vi "POSITION ARMS.vi"(6 "arm angle table":T1) -> ()   [LabVIEW 2020]
uses:
  Robot Global Data.vi
  <vilib>/Rock Robotics/Network Tables/NT Read Number.vi
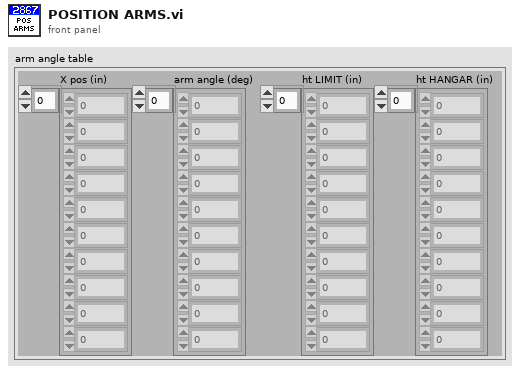
[diagram p1: front panel]
types:
  T1 = cluster{"X pos (in)":dbl[], "arm angle (deg)":dbl[], "ht LIMIT (in)":dbl[], "ht HANGAR (in)":dbl[]}
  T2 = cluster{"MIN":dbl, "MAX":dbl, "convert climber inches to tics":dbl}
  T3 = cluster{"MIN":dbl, "MAX":dbl, "convert arm inches to revs":dbl}
  T4 = typedef "WPI_MotorControlDeviceRef.ctl" = cluster{"DeviceStatus":errorcluster, "Type":T5, "PWM":cluster{"PWM Channel":T6, "DeadBand":T7}, "CAN":cluster{"Device Number":u8, "SetOutput VI Ref":variant, "GetOutput VI Ref":variant, "Enable VI Ref":variant, "Disable VI Ref":variant, "Data":variant}, "Invert":bool, "DIO PWM":cluster{"PWM \"Enable\" Channel":T6, "DIOChannel":T8, "PWM Rate":dbl}}
  T5 = typedef "WPI_MotorControlType.ctl" = enum16{"PWM", "CAN", "DIO PWM"}
  T6 = typedef "FPGA_DIOPWMChannel.ctl" = enum8{"PWM 0", "PWM 1", "PWM 2", "PWM 3", "PWM 4", "PWM 5", "PWM 6", "PWM 7", "PWM 8", "PWM 9", "PWM MXP 0", "PWM MXP 1", "PWM MXP 2", "PWM MXP 3", "PWM MXP 4", "PWM MXP 5", "PWM MXP 6", "PWM MXP 7", "PWM MXP 8", "PWM MXP 9", "Invalid"}
  T7 = typedef "WPI_PWMDeadband.ctl" = cluster{"Name":string, "maxPositivePwm":i32, "minPositivePwm":i32, "centerPwm":i32, "maxNegativePwm":i32, "minNegativePwm":i32, "angularRange":u16}
  T8 = typedef "FPGA_DIOChannel.ctl" = enum8{"DIO 0", "DIO 1", "DIO 2", "DIO 3", "DIO 4", "DIO 5", "DIO 6", "DIO 7", "DIO 8", "DIO 9", "DIO MXP 0", "DIO MXP 1", "DIO MXP 2", "DIO MXP 3", "DIO MXP 4", "DIO MXP 5", "DIO MXP 6", "DIO MXP 7", "DIO MXP 8", "DIO MXP 9", "DIO MXP 10", "DIO MXP 11", "DIO MXP 12", "DIO MXP 13", "DIO MXP 14", "DIO MXP 15", "SPI Port CS1", "SPI Port CS2", "SPI Port CS3", "SPI Port MISO", "SPI Port MOSI", "Invalid"}
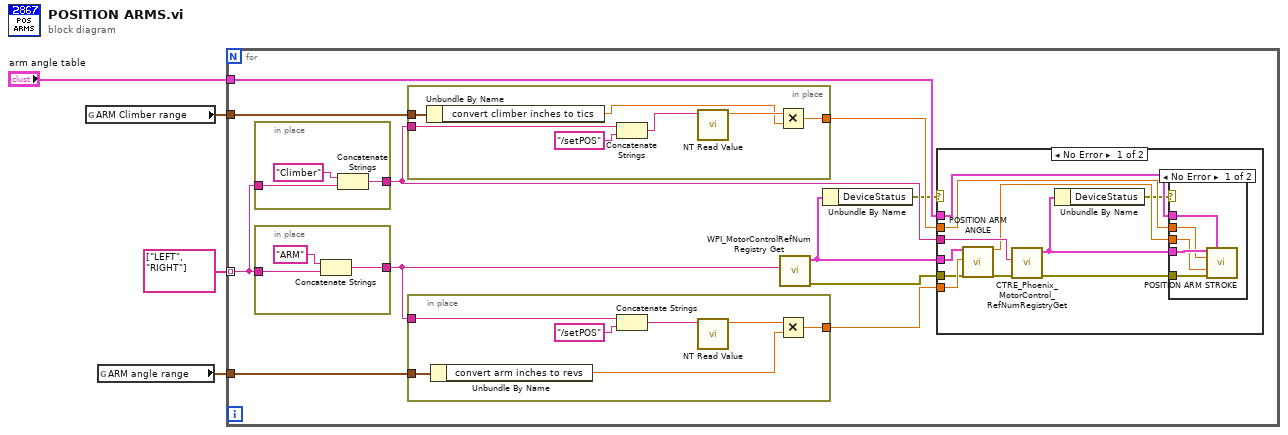
[diagram p0: block diagram]
diagram:
  n1 = global read "Robot Global Data.vi" "ARM Climber range"() -> (w2:T2)
  n2 = global read "Robot Global Data.vi" "ARM angle range"() -> (w1:T3)
  n3 = for {
    tunnel: string[] ["LEFT", "RIGHT"] -> [w12] mode=indexing
    tunnel: "arm angle table" -> [w9]
    tunnel: w2 -> [w8]
    tunnel: w1 -> [w7]
    n4 = in-place {
      in-place-border: [w41] -> w11
      in-place-border: w12 -> [w39]
      n5 = Concatenate Strings("Climber" ("string"), w39) -> (w41:string)
    }
    n6 = in-place {
      in-place-border: [w51] -> w13
      in-place-border: w12 -> [w49]
      n7 = Concatenate Strings("ARM" ("string"), w49) -> (w51:string)
    }
    n8 = in-place {
      in-place-border: [w34] -> w10
      in-place-border: w11 -> [w36]
      in-place-border: w8 -> [w35]
      n9 = Unbundle By Name(w35) -> ("convert climber inches to tics"=w32:dbl)
      n10 = Concatenate Strings(w36, "/setPOS" ("string")) -> (w38:string)
      n11 = call-poly <vilib>:"NT Read Value.vi"("Name"=w38) -> ("Numeric"=w33:dbl)  [unwired: 9 in, 1 out]
      n12 = Multiply(x=w33, y=w32) -> (x*y=w34:dbl)
    }
    n13 = in-place {
      in-place-border: [w43] -> w15
      in-place-border: w13 -> [w47]
      in-place-border: w7 -> [w44]
      n14 = Unbundle By Name(w44) -> ("convert arm inches to revs"=w42:dbl)
      n15 = Concatenate Strings(w47, "/setPOS" ("string")) -> (w46:string)
      n16 = call-poly <vilib>:"NT Read Value.vi"("Name"=w46) -> ("Numeric"=w48:dbl)  [unwired: 9 in, 1 out]
      n17 = Multiply(x=w48, y=w42) -> (x*y=w43:dbl)
    }
    n18 = call <vilib>:"WPI_MotorControlRefNum Registry Get.vi"("refnum name"=w13) -> ("error out"=w14:errorcluster, "MotorControlDevRef"=w5:T4)  [unwired: 9 in]
    n19 = Unbundle By Name(w5) -> ("DeviceStatus"=w6:errorcluster)
    n20 = case shown="No Error" w6 {
      tunnel: w5 -> [w26 _]
      tunnel: w15 -> [w25 _]
      tunnel: w14 -> [w24 _]
      tunnel: w11 -> [w23 _]
      tunnel: w10 -> [w21 _]
      tunnel: w9 -> [w18 _]
      frame No Error {
        n21 = call "POSITION ARM ANGLE.vi"("ARM devref in"=w26, "Setpoint"=w25, "error in (no error)"=w24) -> ("Position"=w20:dbl, "error out"=w22:errorcluster)  [unwired: 14 in, 1 out]
        n22 = call <vilib>:"CTRE_Phoenix_MotorControl_RefNumRegistryGet.vi"("error in (no error)"=w22, "refnum name"=w23) -> ("error out"=w19:errorcluster, "PhoenixMotorControlDevRef"=w16:T4)  [unwired: 8 in]
        n23 = Unbundle By Name(w16) -> ("DeviceStatus"=w17:errorcluster)
        n24 = case shown="No Error" w17 {
          tunnel: w16 -> [w31 _]
          tunnel: w21 -> [w30 _]
          tunnel: w20 -> [w29 _]
          tunnel: w19 -> [w28 _]
          tunnel: w18 -> [w27 _]
          frame No Error {
            n25 = call "POSITION ARM STROKE.vi"("PhoenixMotorControlDevRef"=w31, "arm angle table"=w27, "target position (tics)"=w30, "arm angle motor pos"=w29, "error in (no error)"=w28) -> ()  [unwired: 9 in, 2 out]
          }
          frame Error {
          }
        }
      }
      frame Error {
      }
    }
  }
